vi "PORT IO Write Word__ogtk.vi"(4 "error in (no error)":errorcluster, 5 "fast (F)":bool, 6 "value":u16, 7 "address":u16 format="%.0x") -> (0 "error out":errorcluster)   [LabVIEW 2017]
doc: "This function writes a single word to the specified IO port. If you set fast to True, and are running under Windows NT/2000/XP/2003 you must have enabled the according IO port with a call to \"PORT IO Enable Range.vi\" to avoid a General Protection Fault error."
uses:
  <userlib>/_OpenG.lib/portio/ogportio.dll
panel:
  # "PORT IO Write Word.vi\n\nWrites a word to the port IO range.\n\nPlease visit http://www.OpenG.org to learn about the\nOpen Source LabVIEW software movement.\n\nNOTICE -- YOU MUST LEAVE THIS NOTICE IN PLACE.  PER THE TERMS OF THE LICENSE BELOW, YOU MAY SUBLICENSE THIS SOFTWARE \nIN ANY WAY THAT DOES NOT CONFLICT WITH THIS LICENSE.\n\n### BSD License (http://www.opensource.org/licenses/bsd-license.php) Begin ###\n\nCopyright (c) 2002-2007, Rolf Kalbermatter <rolf.kalbermatter@citeng.com> \n\nAll rights reserved.\n\nRedistribution and use in source and binary forms, with or without modification, are permitted provided that the following conditions are met:\n\n    * Redistributions of source code must retain the above copyright notice, this list of conditions and the following disclaimer.\n    * Redistributions in binary form must reproduce the above copyright notice, this list of conditions and the following disclaimer in the \n       documentation and/or other materials provided with the distribution.\n    * Neither the name of SciWare, James Kring, Inc., nor the names of its contributors may be used to endorse or promote products derived \n       from this software without specific prior written permission.\n\nTHIS SOFTWARE IS PROVIDED BY THE COPYRIGHT HOLDERS AND CONTRIBUTORS \"AS IS\" AND ANY EXPRESS OR IMPLIED WARRANTIES, \nINCLUDING, BUT NOT LIMITED TO, THE IMPLIED WARRANTIES OF MERCHANTABILITY AND FITNESS FOR A PARTICULAR PURPOSE ARE \nDISCLAIMED. IN NO EVENT SHALL THE COPYRIGHT OWNER OR CONTRIBUTORS BE LIABLE FOR ANY DIRECT, INDIRECT, INCIDENTAL,\n SPECIAL, EXEMPLARY, OR CONSEQUENTIAL DAMAGES (INCLUDING, BUT NOT LIMITED TO, PROCUREMENT OF SUBSTITUTE GOODS OR \nSERVICES; LOSS OF USE, DATA, OR PROFITS; OR BUSINESS INTERRUPTION) HOWEVER CAUSED AND ON ANY THEORY OF LIABILITY, \nWHETHER IN CONTRACT, STRICT LIABILITY, OR TORT (INCLUDING NEGLIGENCE OR OTHERWISE) ARISING IN ANY WAY OUT OF THE USE \nOF THIS SOFTWARE, EVEN IF ADVISED OF THE POSSIBILITY OF SUCH DAMAGE.\n\n### BSD License End ###"
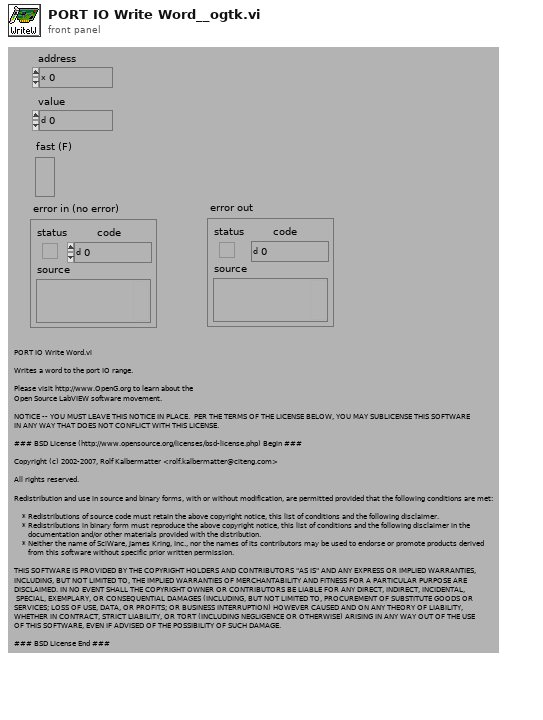
[diagram p1: front panel]
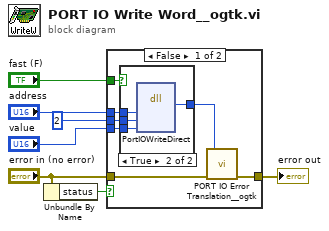
[diagram p0: block diagram]
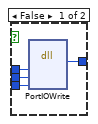
[diagram p2: hidden frame]
diagram:
  n1 = Unbundle By Name("error in (no error)") -> ("status"=w7:bool)
  n2 = case shown="False" w7 {
    tunnel: "error in (no error)" -> [w9 w23]
    tunnel: "address" -> [w13 _]
    tunnel: "value" -> [w12 _]
    tunnel: u32 2 ("process") -> [w11 _]
    tunnel: "fast (F)" -> [w10 _]
    tunnel: [w8 w23] -> w2
    frame False {
      n3 = case shown="True" w10 {
        tunnel: [w15 w22] -> w14
        tunnel: w13 -> [w16 w21]
        tunnel: w12 -> [w18 w20]
        tunnel: w11 -> [w17 w19]
        frame False {
          n4 = dll-call lib="C:/Program Files (x86)/National Instruments/LabVIEW 2017/user.lib/_OpenG.lib/portio/ogportio.*" fn="PortIOWrite"("address"=w16, "size"=w17, "value"=w18) -> (w15:u32)  [unwired: 6 in, 2 out]
        }
        frame True {
          n5 = dll-call lib="C:/Program Files (x86)/National Instruments/LabVIEW 2017/user.lib/_OpenG.lib/portio/ogportio.*" fn="PortIOWriteDirect"("address"=w21, "size"=w19, "value"=w20) -> (w22:u32)  [unwired: 6 in, 2 out]
        }
      }
      n6 = call <userlib>:"PORT IO Error Translation__ogtk.vi"("error in (no error)"=w9, "win error"=w14) -> ("error out"=w8:errorcluster)  [unwired: 5 in]
    }
    frame True {
    }
  }
  "error out" <- w2
